vi "Text1000.vi"   [LabVIEW 2013]
uses:
  <vilib>/Heliosphere Research LLC/Advanced Plotting Toolkit/Advanced Plotting Toolkit.lvlib
types:
  T1 = typedef "Advanced Plotting Toolkit.lvlib/PlotID.ctl" = i32
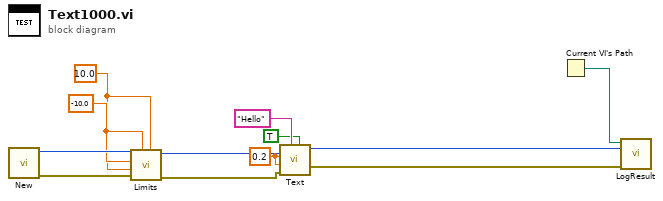
[diagram p0: block diagram]
diagram:
  w2 = 10.0 ("X Max")
  w3 = -10.0 ("X Min")
  w11 = 0.2 ("X Position")
  n1 = call <vilib>:"New.vi"() -> ("error out"=w5:errorcluster, "Plot ID"=w7:T1)  [unwired: 10 in]
  n2 = call <vilib>:"Limits.vi"("Y Max"=w2, "Y Min"=w3, "error in (no error)"=w5, "X Max"=w2, "X Min"=w3, "Plot ID"=w7) -> ("error out"=w4:errorcluster, "Plot ID Out"=w6:T1)  [unwired: 4 in]
  n3 = call <vilib>:"Text.vi"("Relative Coordinates"=TRUE, "Text"="Hello", "error in (no error)"=w4, "Y Position"=w11, "X Position"=w11, "Plot ID"=w6) -> ("error out"=w8:errorcluster, "Plot ID Out"=w9:T1)  [unwired: 4 in]
  n4 = Current VI's Path() -> (path=w12:path)
  n5 = call "LogResult.vi"("Test Result"=w8, "Test Artifact"=w9, "VI Path"=w12) -> ()  [unwired: 9 in]
